vi "经纬度距离计算.vi"(10 "结束位置":cluster{"经度":dbl, "纬度":dbl}, 11 "起始位置":cluster{"经度":dbl, "纬度":dbl}) -> (3 "距离":dbl)   [LabVIEW 2016, in "动力环境.lvlib"]
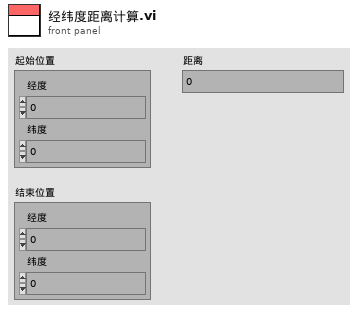
[diagram p1: front panel]
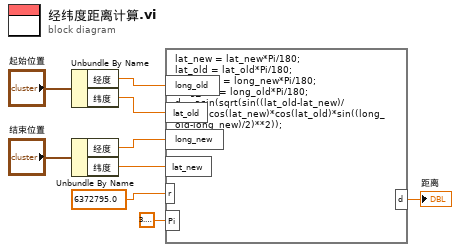
[diagram p0: block diagram]
diagram:
  n1 = Unbundle By Name("起始位置") -> ("经度"=w5:dbl, "纬度"=w4:dbl)
  n2 = Unbundle By Name("结束位置") -> ("经度"=w2:dbl, "纬度"=w1:dbl)
  n3 = formula code="lat_new = lat_new*Pi/180;\nlat_old = lat_old*Pi/180;\nlong_new = long_new*Pi/180;\nlong_old = long_old*Pi/180;\nd = asin(sqrt(sin((lat_old-lat_new)/2)**2+cos(lat_new)*cos(lat_old)*sin((long_old-long_new)/2)**2));\nd = 2*d*r;"("Pi"=3.141592653589793, "r"=6372795.0, "long_old"=w5, "long_new"=w2, "lat_old"=w4, "lat_new"=w1) -> ("d"=→"距离":dbl)
